vi "Average_Block_Timetraces.vi"() -> (5 "Plug in titles":string[](array[string]), 7 "Plug in values":string[](array[string]))   [LabVIEW 2011]
uses:
  Globals/Meas_global.vi
panel:
  out "XY Graph":cluster{"Time (ms)":dbl[], dbl[]}(graph)
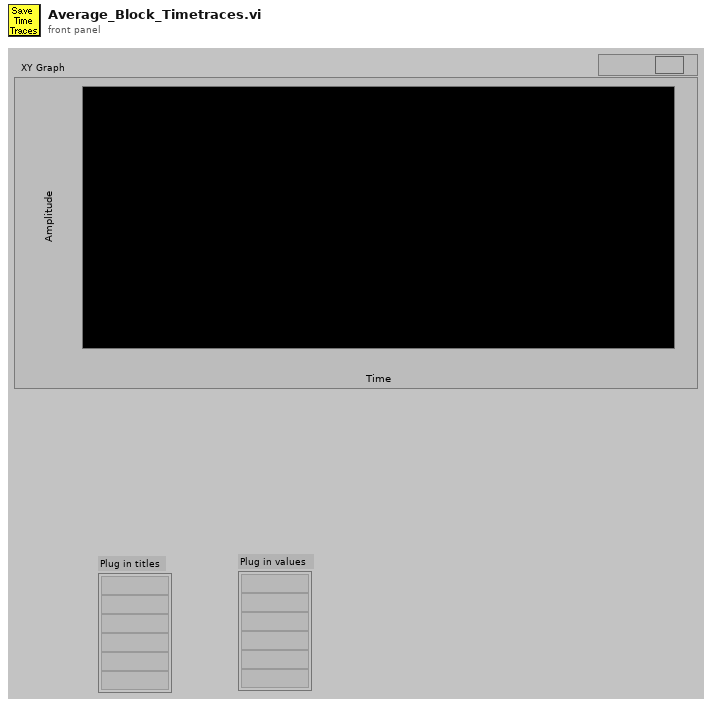
[diagram p1: front panel]
types:
  T1 = typedef "Analysis_info_cluster.ctl" = cluster{"Colour":u32, "Inst type":T2, "Inst name":string, "Symbol":string, "Code name":string, "Extra Info":string, "Inst Array":T3, "Extra Titles":string[], "Extra Values":string[], "Eng Values":dbl[], "Time (ms)":dbl[], "Voltage":dbl[], "U":dbl, "u^2":dbl, "u^3":dbl, "u^4":dbl, "Skew_u":dbl, "Kurt_u":dbl, "Sd Error in Mean":dbl, "% u'/U":dbl, "X":dbl, "Y":dbl, "Z":dbl, "Spectra":T4, "Autocorrelation":T4, "Timescale integral to 25%":dbl, "Sd Error in Variance":dbl, "Calib File":path, "Calib Constants":dbl[], "Histogram":T4, "Output Position":bool, "Full Stats":bool, "Weighting":dbl[], "Av Sampling Rate":dbl, "Av No of Samples":dbl, "Total Meas Time (s)":dbl}
  T2 = typedef "Inst_type.ctl" = enum16{"Propeller anemometer", "Raw voltage", "Pressure Transducer", "Pitot-static tube", "Preston tube", "Hot wire", "Cross wire 1", "Cross wire 2", "Generic Linear", "Generic Polynomial", "Generic BackPoly", "Fast FID", "Thermocouple", "Cold wire", "Pulsed Wire", "LDA Vel", "LDA Tran time", "LDA Arr time"}
  T3 = typedef "Instrument_Array.ctl" = enum16{"PWA", "LDA", "Analogue"}
  T4 = typedef "XY_Plot_Cluster.ctl" = cluster{"First Name":string, "Second Name":string, "X axis name":string, "Y axis name":string, "X array":dbl[], "Y array":dbl[]}
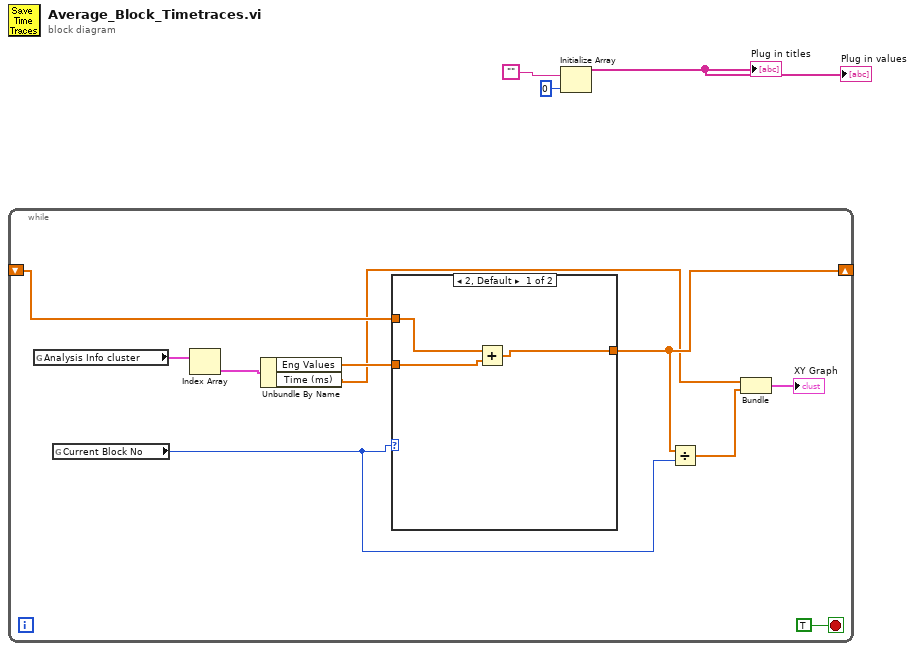
[diagram p0: block diagram]
diagram:
  n1 = while {
    shift-right: [w9] -> _
    shift-left: _ -> [w10]
    stop <- TRUE stop-if-true
    n2 = global read "Meas_global.vi" "Analysis Info cluster"() -> (w13:T1[])
    n3 = global read "Meas_global.vi" "Current Block No"() -> (w8:i32)
    n4 = Index Array(array=w13) -> (element=w12:T1)  [unwired: 1 in]
    n5 = Unbundle By Name(w12) -> ("Eng Values"=w11:dbl[], "Time (ms)"=w7:dbl[])
    n6 = case shown="2, Default" w8 {
      tunnel: [w14 w17] -> w9
      tunnel: w11 -> [w16 w17]
      tunnel: w10 -> [w15 _]
      frame 2, Default {
        n7 = Add(x=w15, y=w16) -> (x+y=w14:dbl[])
      }
      frame 1 {
      }
    }
    n8 = Divide(x=w9, y=w8) -> (x/y=w6:dbl[])
    n9 = Bundle("Time (ms)"=w7, w6) -> (→"XY Graph":cluster{"Time (ms)":dbl[], dbl[]})  [unwired: 1 in]
  }
  n10 = Initialize Array("", 0) -> (→"Plug in values" →"Plug in titles":string[])
